vi "Set Raw Header.vi"(8 "error in (no error)":errorcluster, 10 "Header":string, 11 "Request in":refnum<class "Request.lvclass">) -> (0 "error out":errorcluster, 3 "Request out":refnum<class "Request.lvclass">)   [LabVIEW 2017, in "Request.lvclass"]
uses:
  Request.lvclass
  Request.lvclass/Request.ctl
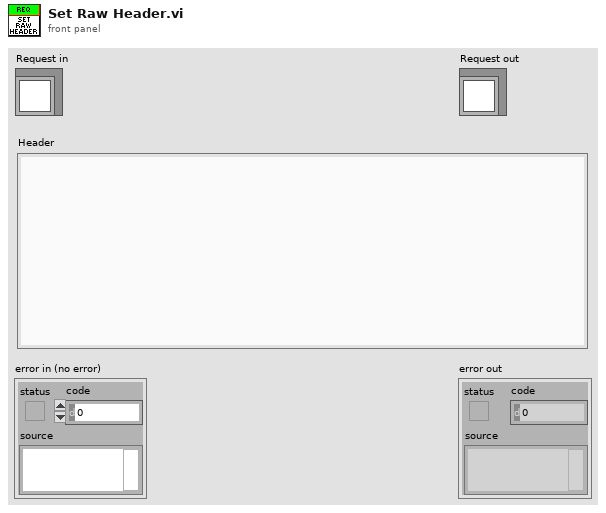
[diagram p1: front panel]
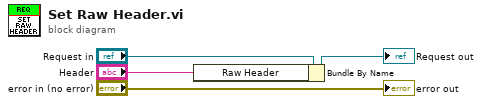
[diagram p0: block diagram]
diagram:
  n1 = Bundle By Name(cluster="Request in", "Raw Header"="Header") -> (→"Request out":refnum<class "Request.lvclass">)
  "error out" <- "error in (no error)"
